vi "Save Measurement File.vi"(0 "Measurement Save Path":path, 1 "Measurement Type":T2, 2 "Data in (if 1D)":i64[](array[numeric]), 3 "Data in (if 2D)":u16[][](array[numeric]), 4 "mesh":i32, 5 "ND angle":u32, 6 "tac":i32, 7 "Position":dbl[](array[numeric]), 8 "x center":i32, 9 "y center":i32, 10 "gain":i32, 11 "integration time":i32, 12 "bins":i32, 13 "Filename Note":string, 14 "Filter":string, 15 "x range":i32, 16 "y range":i32, 18 "image data":T1, 19 "laser power":i32) -> ()   [LabVIEW 2023]
uses:
  MeasurementType.ctl
  <vilib>/picture/picture.llb/imagedata.ctl
  <vilib>/Utility/file.llb/Write Delimited Spreadsheet (I64).vi
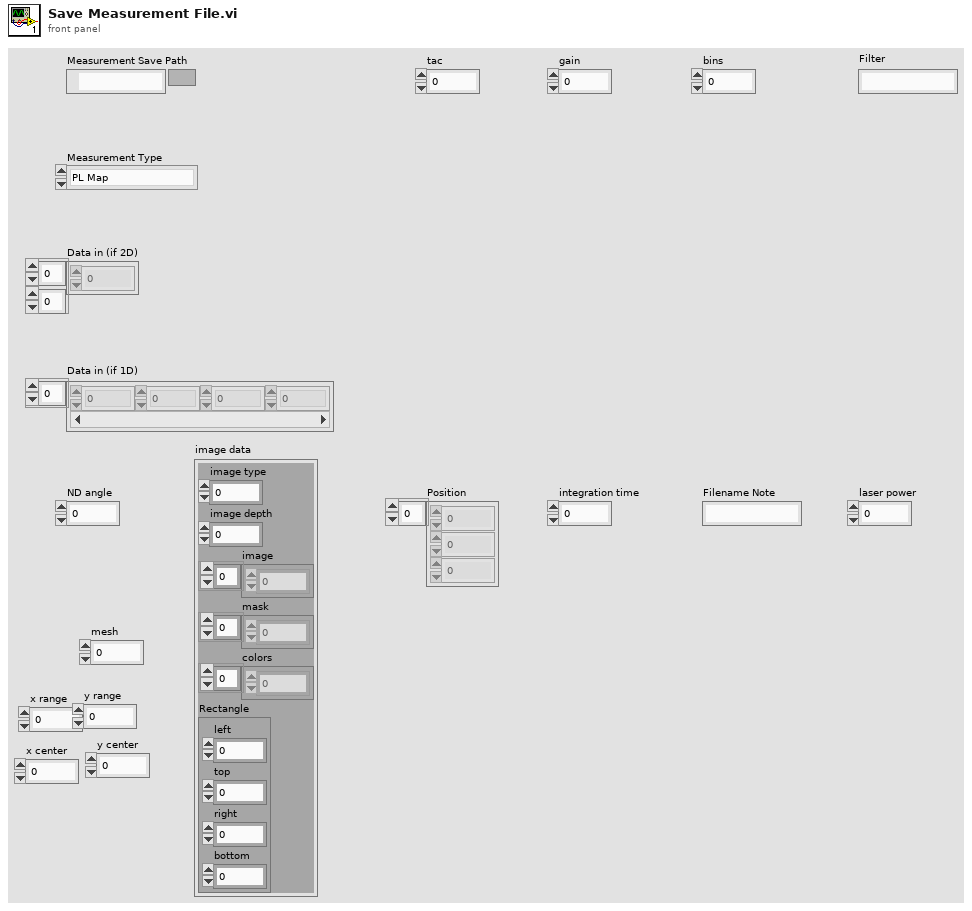
[diagram p1: front panel]
types:
  T1 = typedef "imagedata.ctl" = cluster{"image type":i32, "image depth":i32, "image":u8[], "mask":u8[], "colors":u32[], "Rectangle":cluster{"left":i16, "top":i16, "right":i16, "bottom":i16}}
  T2 = typedef "MeasurementType.ctl" = enum16{"PL Map", "Spectrum", "Lifetime", "g2", "Stability", "Saturation"}
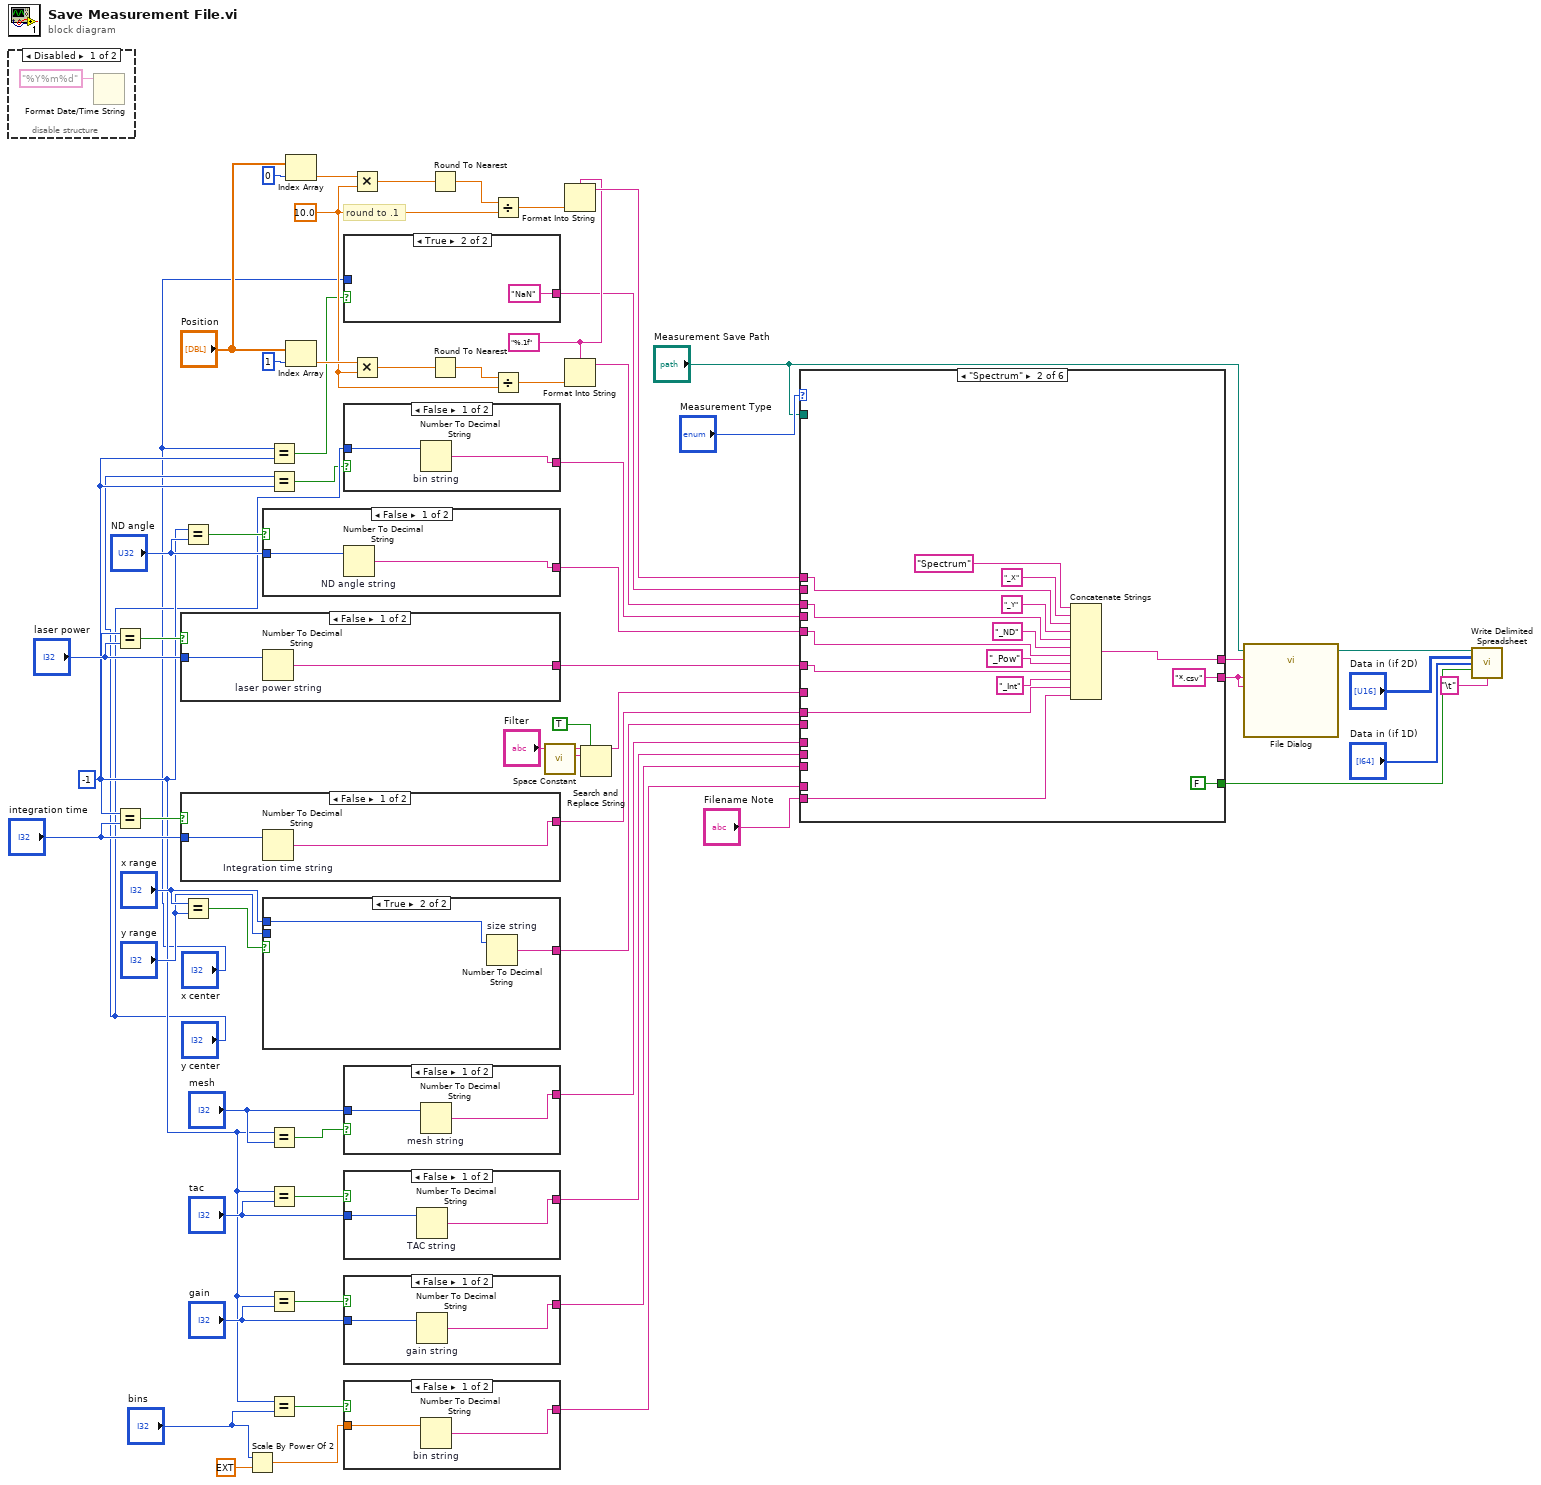
[diagram p0: block diagram]
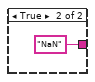
[diagram p2: hidden frame]
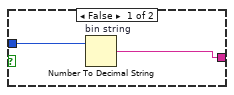
[diagram p3: hidden frame]
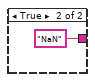
[diagram p4: hidden frame]
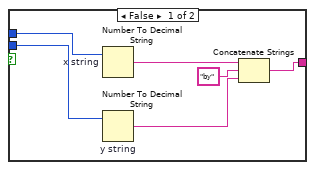
[diagram p5: hidden frame]
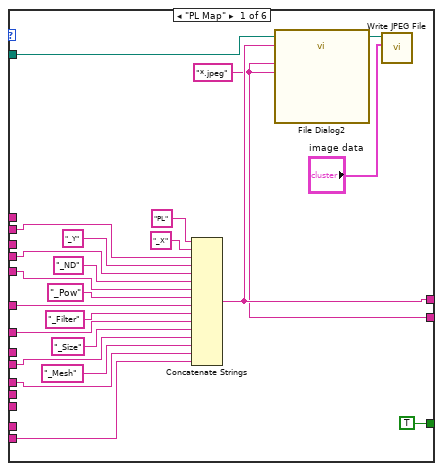
[diagram p6: hidden frame]
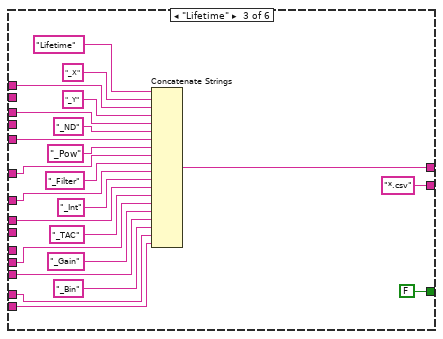
[diagram p7: hidden frame]
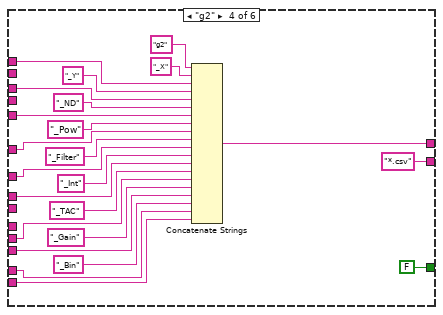
[diagram p8: hidden frame]
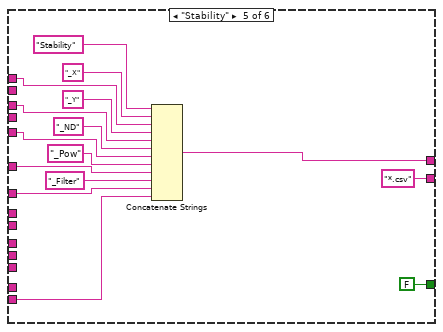
[diagram p9: hidden frame]
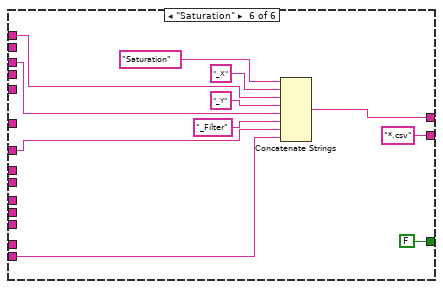
[diagram p10: hidden frame]
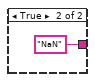
[diagram p12: hidden frame]
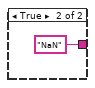
[diagram p13: hidden frame]
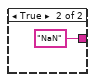
[diagram p14: hidden frame]
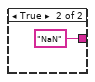
[diagram p15: hidden frame]
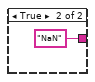
[diagram p16: hidden frame]
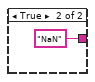
[diagram p17: hidden frame]
diagram:
  w28 = "%.1f" ("format string")
  w10 = -1 ("x")
  w50 = 10.0 ("y")
  # "round to .1"
  n1 = disable-structure shown="Disabled" {
    frame Disabled {
      n2 = Format Date/Time String(time format string (%c)="%Y%m%d") -> ()  [unwired: 2 in, 1 out]
    }
    frame Enabled {
    }
  }
  n3 = Equal?(x=w10, y="laser power") -> (x = y?=w42:bool)
  n4 = Equal?(x=w10, y="integration time") -> (x = y?=w49:bool)
  n5 = case shown="False" w42 {
    tunnel: "laser power" -> [w66 _]
    tunnel: [w65 "NaN"] -> w37
    frame False {
      n6 = Number To Decimal String "laser power string"(number=w66) -> (decimal integer string=w65:string)  [unwired: 1 in]
    }
    frame True {
    }
  }
  n7 = case shown="False" w49 {
    tunnel: [w68 "NaN"] -> w35
    tunnel: "integration time" -> [w69 _]
    frame False {
      n8 = Number To Decimal String "Integration time string"(number=w69) -> (decimal integer string=w68:string)  [unwired: 1 in]
    }
    frame True {
    }
  }
  n9 = Equal?(x=w10, y="ND angle") -> (x = y?=w43:bool)
  n10 = Equal?(x="x range", y="y range") -> (x = y?=w17:bool)
  n11 = Scale By Power Of 2(n="bins", x=ext 1.0) -> (x*2^n=w1:ext)
  n12 = case shown="False" w43 {
    tunnel: [w71 "NaN"] -> w40
    tunnel: "ND angle" -> [w72 _]
    frame False {
      n13 = Number To Decimal String "ND angle string"(number=w72) -> (decimal integer string=w71:string)  [unwired: 1 in]
    }
    frame True {
    }
  }
  n14 = case shown="True" w17 {
    tunnel: "x range" -> [w79 w81]
    tunnel: "y range" -> [w78 _]
    tunnel: [w77 w80] -> w11
    frame False {
      n15 = Number To Decimal String "x string"(number=w79) -> (decimal integer string=w76:string)  [unwired: 1 in]
      n16 = Number To Decimal String "y string"(number=w78) -> (decimal integer string=w74:string)  [unwired: 1 in]
      n17 = Concatenate Strings(w76, "by", w74) -> (w77:string)
    }
    frame True {
      n18 = Number To Decimal String "size string"(number=w81) -> (decimal integer string=w80:string)  [unwired: 1 in]
    }
  }
  n19 = Equal?(x="x center", y=w10) -> (x = y?=w7:bool)
  n20 = Equal?(x="y center", y=w10) -> (x = y?=w8:bool)
  n21 = Equal?(x=w10, y="mesh") -> (x = y?=w14:bool)
  n22 = Equal?(x=w10, y="tac") -> (x = y?=w45:bool)
  n23 = Equal?(x=w10, y="gain") -> (x = y?=w46:bool)
  n24 = Equal?(x=w10, y="bins") -> (x = y?=w47:bool)
  n25 = Index Array(array="Position", index=0) -> (element=w56:dbl)
  n26 = Index Array(array="Position", index=1) -> (element=w53:dbl)
  n27 = case shown="True" w7 {
    tunnel: "x center" -> [w83 _]
    tunnel: [w82 "NaN"] -> w5
    frame False {
      n28 = Number To Decimal String "bin string"(number=w83) -> (decimal integer string=w82:string)  [unwired: 1 in]
    }
    frame True {
    }
  }
  n29 = case shown="False" w8 {
    tunnel: "y center" -> [w86 _]
    tunnel: [w85 "NaN"] -> w4
    frame False {
      n30 = Number To Decimal String "bin string"(number=w86) -> (decimal integer string=w85:string)  [unwired: 1 in]
    }
    frame True {
    }
  }
  n31 = case shown="False" w14 {
    tunnel: "mesh" -> [w89 _]
    tunnel: [w88 "NaN"] -> w13
    frame False {
      n32 = Number To Decimal String "mesh string"(number=w89) -> (decimal integer string=w88:string)  [unwired: 1 in]
    }
    frame True {
    }
  }
  n33 = case shown="False" w45 {
    tunnel: [w91 "NaN"] -> w39
    tunnel: "tac" -> [w92 _]
    frame False {
      n34 = Number To Decimal String "TAC string"(number=w92) -> (decimal integer string=w91:string)  [unwired: 1 in]
    }
    frame True {
    }
  }
  n35 = case shown="False" w46 {
    tunnel: "gain" -> [w95 _]
    tunnel: [w94 "NaN"] -> w36
    frame False {
      n36 = Number To Decimal String "gain string"(number=w95) -> (decimal integer string=w94:string)  [unwired: 1 in]
    }
    frame True {
    }
  }
  n37 = case shown="False" w47 {
    tunnel: w1 -> [w98 _]
    tunnel: [w97 "NaN"] -> w38
    frame False {
      n38 = Number To Decimal String "bin string"(number=w98) -> (decimal integer string=w97:string)  [unwired: 1 in]
    }
    frame True {
    }
  }
  n39 = Multiply(x=w56, y=w50) -> (x*y=w55:dbl)
  n40 = Multiply(x=w53, y=w50) -> (x*y=w54:dbl)
  n41 = Round To Nearest(number=w55) -> (nearest integer value=w52:dbl)
  n42 = Round To Nearest(number=w54) -> (nearest integer value=w51:dbl)
  n43 = Divide(x=w52, y=w50) -> (x/y=w31:dbl)
  n44 = Divide(x=w51, y=w50) -> (x/y=w29:dbl)
  n45 = call <vilib>:"Space Constant.vi"() -> ("String"=w24:string)
  n46 = Format Into String(format string=w28, w31) -> (resulting string=w30:string)  [unwired: 2 in, 1 out]
  n47 = Format Into String(format string=w28, w29) -> (resulting string=w27:string)  [unwired: 2 in, 1 out]
  n48 = Search and Replace String(replace all?=TRUE ("replace all? (F)"), input string="Filter", search string=w24) -> (result string=w22:string)  [unwired: 5 in, 3 out]
  n49 = case shown="\"Spectrum\"" "Measurement Type" {
    tunnel: [w111 w136 w159 w182 w197 w208] -> w59
    tunnel: "Filename Note" -> [w113 w130 w153 w176 w192 w205]
    tunnel: w40 -> [w103 w129 w149 w172 w191 _]
    tunnel: w39 -> [_ _ w148 w171 _ _]
    tunnel: w38 -> [_ _ w147 w170 _ _]
    tunnel: w37 -> [w104 w128 w146 w169 w190 _]
    tunnel: w36 -> [_ _ w145 w168 _ _]
    tunnel: w35 -> [_ w127 w144 w167 _ _]
    tunnel: w30 -> [_ w126 w143 w166 w189 w204]
    tunnel: w27 -> [_ w124 w142 w165 w188 w203]
    tunnel: w22 -> [w105 _ w140 w163 w186 w201]
    tunnel: [w110 "*.csv" ("pattern label") "*.csv" ("pattern label") "*.csv" ("pattern label") "*.csv" ("pattern label") "*.csv" ("pattern label")] -> w19
    tunnel: "Measurement Save Path" -> [w112 _ _ _ _ _]
    tunnel: [TRUE FALSE FALSE FALSE FALSE FALSE] -> w18
    tunnel: w13 -> [w107 _ _ _ _ _]
    tunnel: w11 -> [w106 _ _ _ _ _]
    tunnel: w5 -> [w101 _ _ _ _ _]
    tunnel: w4 -> [w100 _ _ _ _ _]
    frame "PL Map" {
      w110 = "*.jpeg" ("pattern label")
      n50 = Concatenate Strings("PL" ("string"), "_X", w101, "_Y", w100, "_ND" ("string"), w103, "_Pow", w104, "_Filter" ("string"), w105, "_Size", w106, "_Mesh" ("string"), w107, w113) -> (w111:string)
      n51 = call "File Dialog2"("start path"=w112, "default name"=w111, "pattern (all files)"=w110, "pattern label"=w110) -> ("selected path"=w109:path)  [unwired: 8 in, 3 out]
      n52 = call <vilib>:"Write JPEG File.vi"("image data"="image data", "path to JPEG file"=w109) -> ()  [unwired: 8 in, 2 out]
    }
    frame "Spectrum" {
      n53 = Concatenate Strings("Spectrum" ("string"), "_X", w126, "_Y", w124, "_ND" ("string"), w129, "_Pow", w128, "_Int", w127, w130) -> (w136:string)
    }
    frame "Lifetime" {
      n54 = Concatenate Strings("Lifetime" ("string"), "_X", w143, "_Y", w142, "_ND" ("string"), w149, "_Pow", w146, "_Filter" ("string"), w140, "_Int", w144, "_TAC" ("string"), w148, "_Gain" ("string"), w145, "_Bin" ("string"), w147, w153) -> (w159:string)
    }
    frame "g2" {
      n55 = Concatenate Strings("g2" ("string"), "_X", w166, "_Y", w165, "_ND" ("string"), w172, "_Pow", w169, "_Filter" ("string"), w163, "_Int", w167, "_TAC" ("string"), w171, "_Gain" ("string"), w168, "_Bin" ("string"), w170, w176) -> (w182:string)
    }
    frame "Stability" {
      n56 = Concatenate Strings("Stability" ("string"), "_X", w189, "_Y", w188, "_ND" ("string"), w191, "_Pow", w190, "_Filter" ("string"), w186, w192) -> (w197:string)
    }
    frame "Saturation" {
      n57 = Concatenate Strings("Saturation" ("string"), "_X", w204, "_Y", w203, "_Filter" ("string"), w201, w205) -> (w208:string)
    }
  }
  n58 = call "File Dialog"("start path"="Measurement Save Path", "default name"=w59, "pattern (all files)"=w19, "pattern label"=w19) -> ("selected path"=w60:path)  [unwired: 8 in, 3 out]
  n59 = call-poly <vilib>:"Write Delimited Spreadsheet.vi"("file path (dialog if empty)"=w60, "2D data"="Data in (if 2D)", "1D data"="Data in (if 1D)", "append to file? (new file:F)"=w18, "delimiter (\\t)"="\t" ("delimiter (\\t)")) -> ()  [unwired: 9 in, 2 out]
